vi "test.Create.OrderExecutedAtPrice.vi"(11 "OrderExecutedAtPriceSize.Parameters":T1={"Time Offset"=447000, "Order Id"="ORID0001", "Executed Quantity"=20000, "Execution Id"="AAPL", "Price"=0.905, "Remaining Quantity"=20000}) -> (3 "Passed":bool)   [LabVIEW 2022 SP3]
uses:
  OrderExecuted/OrderExecutedAtPriceSize.Parameters.ctl
  OrderExecuted/OrderExecutedAtPriceSize.lvclass
panel:
  out "x = y?":bool[](array[boolean])
  out "Python.Bytes.Out":u8[](array[numeric]) format="%.0x"
  out "LabVIEW.Bytes.Out":u8[](array[numeric]) format="%.0x"
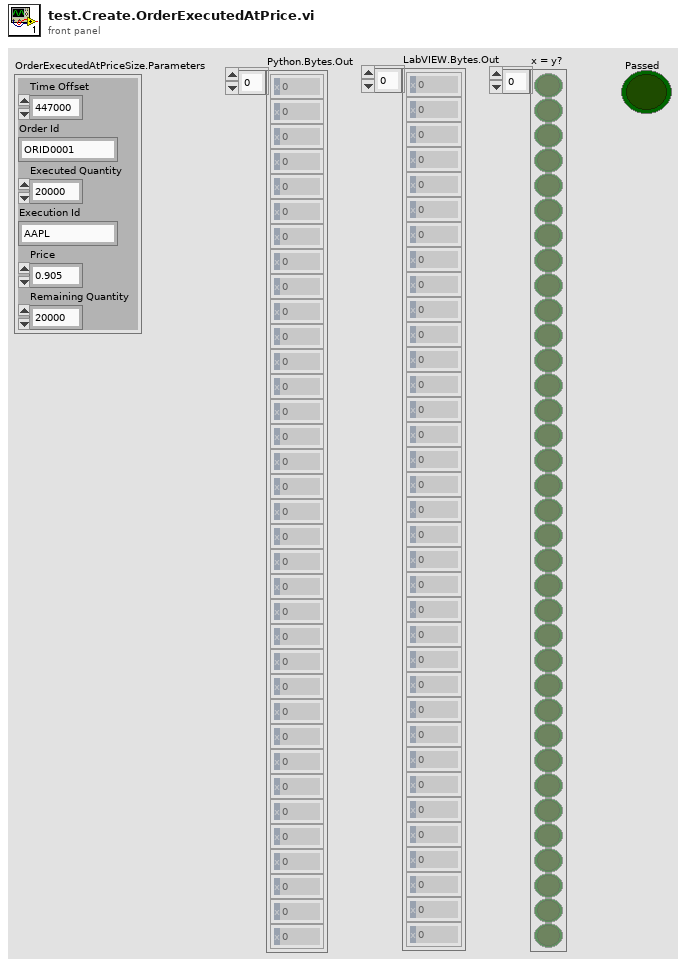
[diagram p1: front panel]
types:
  T1 = typedef "OrderExecutedAtPriceSize.lvclass/OrderExecutedAtPriceSize.Parameters.ctl" = cluster{"Time Offset":u32, "Order Id":string, "Executed Quantity":u32, "Execution Id":string, "Price":dbl, "Remaining Quantity":u32}
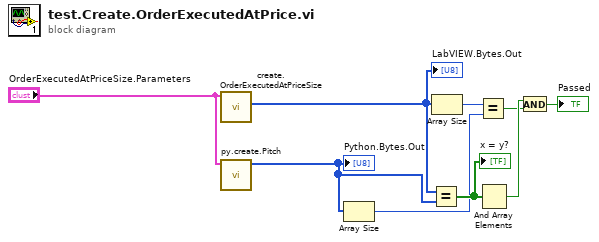
[diagram p0: block diagram]
diagram:
  n1 = call "create.OrderExecutedAtPriceSize.vi"("OrderExecutedAtPriceSize.Parameters"="OrderExecutedAtPriceSize.Parameters") -> ("Bytes.Out"=w6:u8[])  [unwired: 10 in]
  "LabVIEW.Bytes.Out" <- w6
  n2 = call "py.create.Pitch.vi"("Parameters"="OrderExecutedAtPriceSize.Parameters") -> ("bytes"=w5:u8[])  [unwired: 9 in, 1 out]
  "Python.Bytes.Out" <- w5
  n3 = Array Size(array=w5) -> (size(s)=w3:i32)
  n4 = Equal?(x=w6, y=w5) -> (x = y?=w9:bool[])
  "x = y?" <- w9
  n5 = Array Size(array=w6) -> (size(s)=w4:i32)
  n6 = Equal?(x=w4, y=w3) -> (x = y?=w1:bool)
  n7 = And Array Elements(Boolean array=w9) -> (logical AND=w8:bool)
  n8 = And(x=w8, y=w1) -> (x .and. y?=→"Passed":bool)
